vi "Some empty VI 4.vi"(8 "Error In":errorcluster, 10 "StringParam":string, 11 "NumericParam":dbl) -> (0 "Error Out":errorcluster, 3 "String":string="This is just EMPTY VI string which you are supposed to see in generated code.\nTRUE\n     TRUE")   [LabVIEW 2018]
panel:
  out "String 3":string
  out "String 2":string="This is just EMPTY VI string which you are supposed to see in generated code.\nFalse\nFalse\nFalse False False\nFalse"
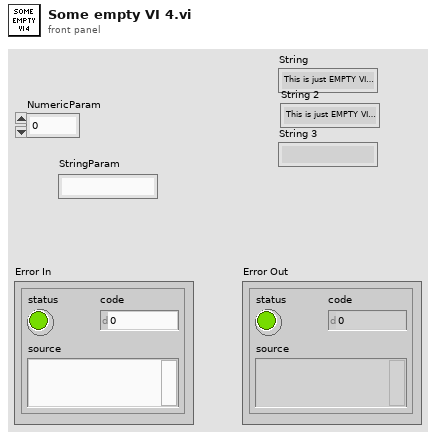
[diagram p1: front panel]
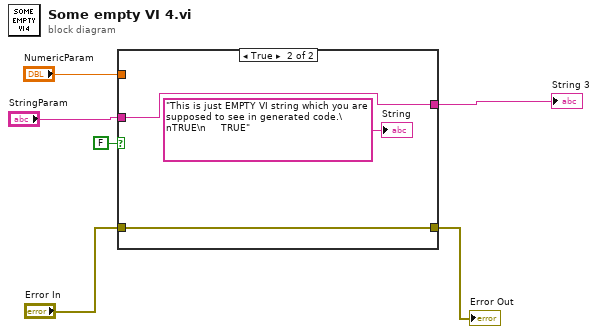
[diagram p0: block diagram]
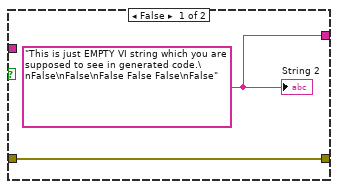
[diagram p2: hidden frame]
diagram:
  n1 = case shown="True" FALSE {
    tunnel: [w8 w11] -> w5
    tunnel: "Error In" -> [w8 w11]
    tunnel: [w7 w9] -> w3
    tunnel: "StringParam" -> [_ w9]
    tunnel: "NumericParam" -> [_ _]
    frame False {
      w7 = "This is just EMPTY VI string which you are supposed to see in generated code.\nFalse\nFalse\nFalse False False\nFalse"
      "String 2" <- w7
    }
    frame True {
      "String" <- "This is just EMPTY VI string which you are supposed to see in generated code.\nTRUE\n     TRUE"
    }
  }
  "Error Out" <- w5
  "String 3" <- w3
